vi "SS_PTF_indexer.vi"(6 "Faults Mod 5":bool[](array[boolean])=[FALSE, FALSE, FALSE], 8 "Faults Mod 4":bool[](array[boolean])=[FALSE, FALSE, FALSE], 9 "Faults Mod 3":bool[](array[boolean])=[FALSE, FALSE, FALSE, FALSE, FALSE, FALSE, FALSE, FALSE, FALSE, FALSE, FALSE, FALSE, FALSE, FALSE, FALSE, FALSE], 10 "Faults Mod 2":bool[](array[boolean])=[FALSE, FALSE, FALSE, FALSE, FALSE, FALSE, FALSE, FALSE, FALSE, FALSE, FALSE, FALSE, FALSE, FALSE, FALSE, FALSE], 11 "Faults Mod 1":bool[](array[boolean])=[FALSE, FALSE, FALSE, FALSE, FALSE, FALSE, FALSE, FALSE, FALSE, FALSE, FALSE, FALSE, FALSE, FALSE, FALSE, FALSE]) -> (3 "Group PTF":bool[](array[boolean]))   [LabVIEW 2016]
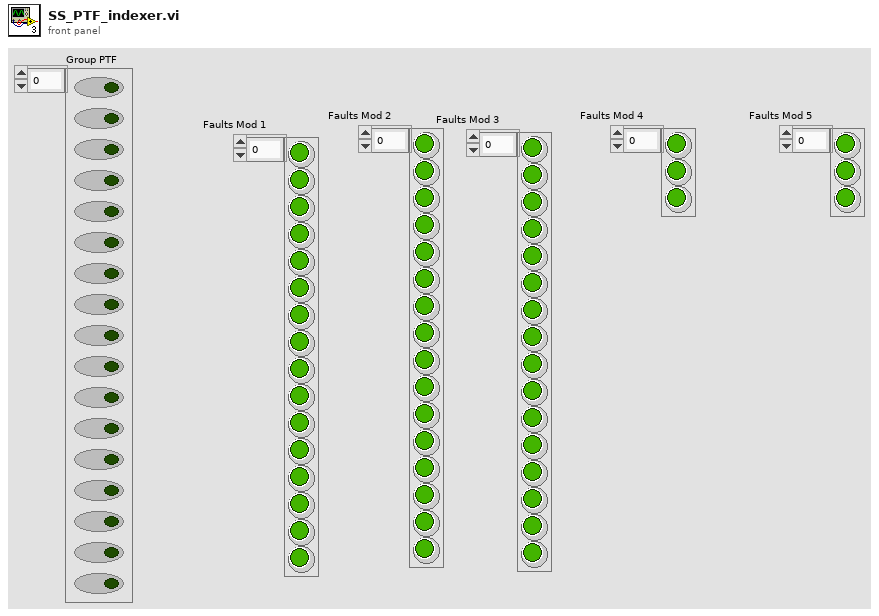
[diagram p1: front panel]
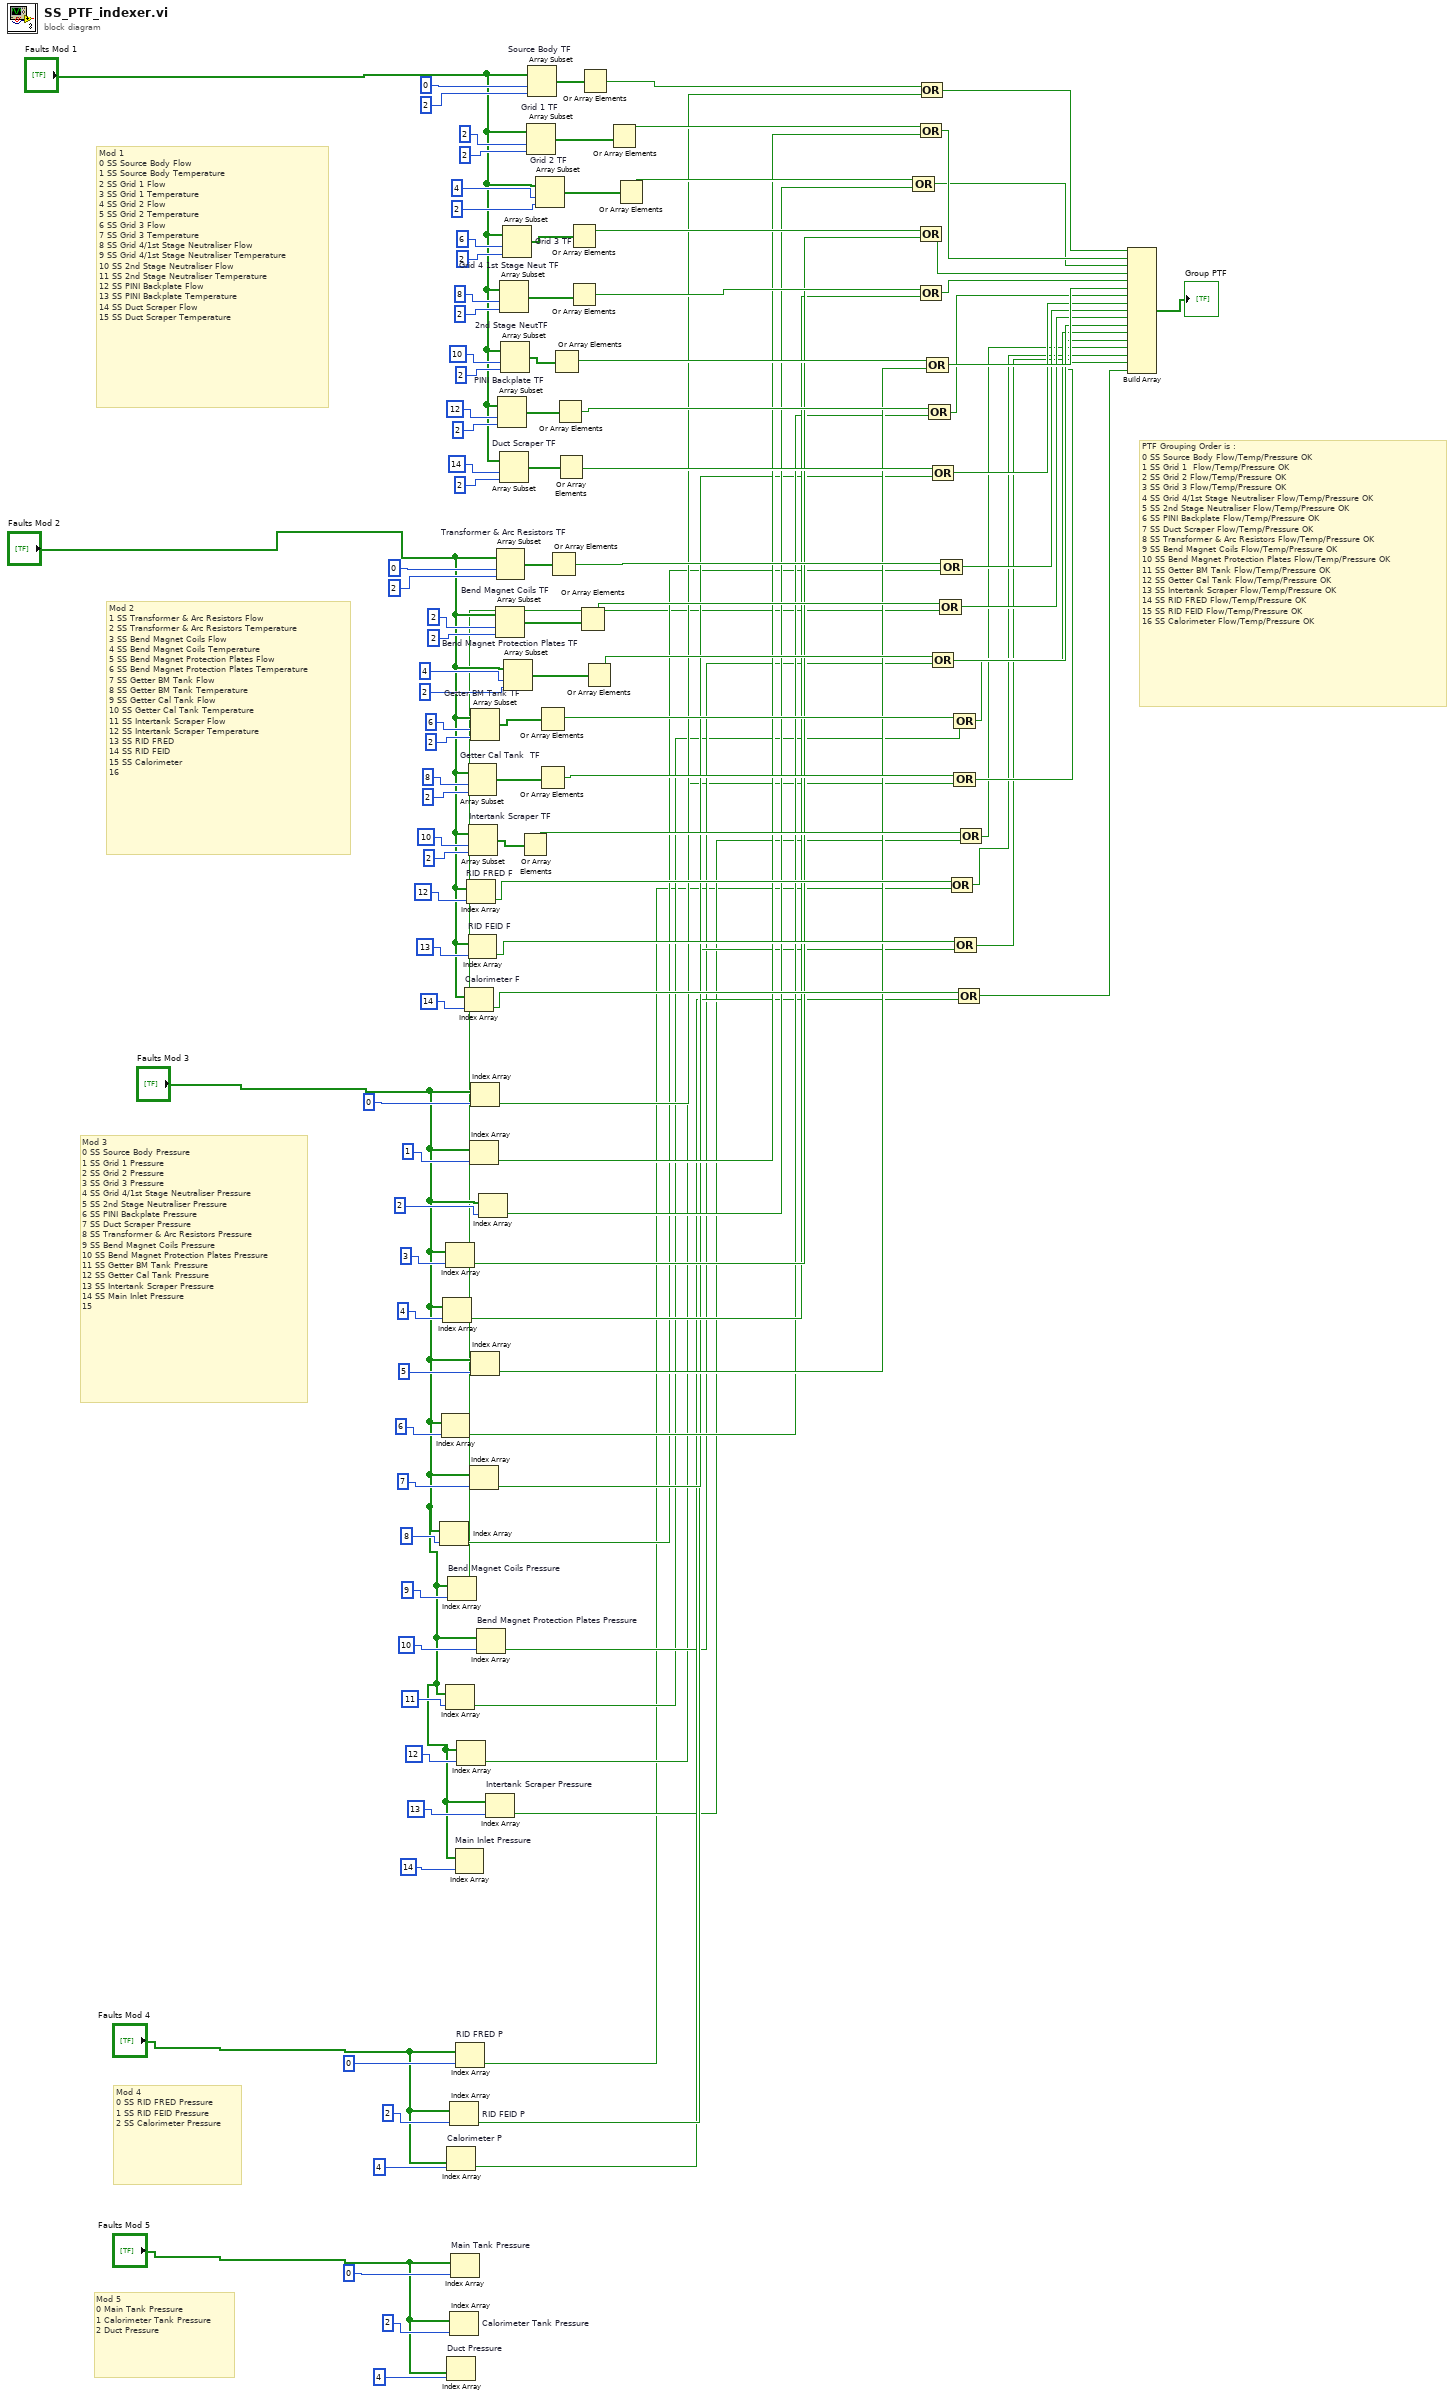
[diagram p0: block diagram]
diagram:
  # "Mod 5\n0\tMain Tank Pressure\n1\tCalorimeter Tank Pressure\n2\tDuct Pressure"
  # "Mod 4\n0\tSS RID FRED Pressure\n1\tSS RID FEID Pressure\n2\tSS Calorimeter Pressure"
  # "Mod 3\n0\tSS Source Body Pressure\n1\tSS Grid 1 Pressure\n2\tSS Grid 2 Pressure\n3\tSS Grid 3 Pressure\n4\tSS Grid 4/1st Stage Neutraliser Pressure\n5\tSS 2nd Stage Neutraliser Pressure\n6\tSS PINI Backplate Pressure\n7\tSS Duct Scraper Pressure\n8\tSS Transformer & Arc Resistors Pressure\n9\tSS Bend Magnet Coils Pressure\n10\tSS Bend Magnet Protection Plates Pressure\n11\tSS Getter BM Tank Pressure\n12\tSS Getter Cal Tank Pressure\n13\tSS Intertank Scraper Pressure\n14\tSS Main Inlet Pressure\n15"
  # "Mod 2\n1\tSS Transformer & Arc Resistors Flow\n2\tSS Transformer & Arc Resistors Temperature\n3\tSS Bend Magnet Coils Flow\n4\tSS Bend Magnet Coils Temperature\n5\tSS Bend Magnet Protection Plates Flow\n6\tSS Bend Magnet Protection Plates Temperature\n7\tSS Getter BM Tank Flow\n8\tSS Getter BM Tank Temperature\n9\tSS Getter Cal Tank Flow\n10\tSS Getter Cal Tank Temperature\n11\tSS Intertank Scraper Flow\n12\tSS Intertank Scraper Temperature\n13\tSS RID FRED\n14\tSS RID FEID\n15\tSS Calorimeter\n16"
  # "Mod 1\n0\tSS Source Body Flow\n1\tSS Source Body Temperature\n2\tSS Grid 1 Flow\n3\tSS Grid 1 Temperature\n4\tSS Grid 2 Flow\n5\tSS Grid 2 Temperature\n6\tSS Grid 3 Flow\n7\tSS Grid 3 Temperature\n8\tSS Grid 4/1st Stage Neutraliser Flow\n9\tSS Grid 4/1st Stage Neutraliser Temperature\n10\tSS 2nd Stage Neutraliser Flow\n11\tSS 2nd Stage Neutraliser Temperature\n12\tSS PINI Backplate Flow\n13\tSS PINI Backplate Temperature\n14\tSS Duct Scraper Flow\n15\tSS Duct Scraper Temperature"
  # "PTF Grouping Order is :\n0\tSS Source Body Flow/Temp/Pressure OK\n1\tSS Grid 1  Flow/Temp/Pressure OK\n2\tSS Grid 2 Flow/Temp/Pressure OK\n3\tSS Grid 3 Flow/Temp/Pressure OK\n4\tSS Grid 4/1st Stage Neutraliser Flow/Temp/Pressure OK\n5\tSS 2nd Stage Neutraliser Flow/Temp/Pressure OK\n6\tSS PINI Backplate Flow/Temp/Pressure OK\n7\tSS Duct Scraper Flow/Temp/Pressure OK\n8\tSS Transformer & Arc Resistors Flow/Temp/Pressure OK\n9\tSS Bend Magnet Coils Flow/Temp/Pressure OK\n10\tSS Bend Magnet Protection Plates Flow/Temp/Pressure OK\n11\tSS Getter BM Tank Flow/Temp/Pressure OK\n12\tSS Getter Cal Tank Flow/Temp/Pressure OK\n13\tSS Intertank Scraper Flow/Temp/Pressure OK\n14\tSS RID FRED Flow/Temp/Pressure OK\n15\tSS RID FEID Flow/Temp/Pressure OK\n16\tSS Calorimeter Flow/Temp/Pressure OK"
  n1 = Index Array "Index Array"(array="Faults Mod 3", index=8) -> (element=w25:bool)
  n2 = Index Array "Index Array"(array="Faults Mod 3", index=6) -> (element=w44:bool)
  n3 = Index Array "Index Array"(array="Faults Mod 3", index=4) -> (element=w46:bool)
  n4 = Index Array "Index Array"(array="Faults Mod 3", index=3) -> (element=w47:bool)
  n5 = Index Array "Index Array"(array="Faults Mod 3", index=11) -> (element=w22:bool)
  n6 = Index Array "Calorimeter P"(array="Faults Mod 4", index=4) -> (element=w37:bool)
  n7 = Index Array "Duct Pressure"(array="Faults Mod 5", index=4) -> ()  [unwired: 1 out]
  n8 = Index Array "Bend Magnet Coils Pressure"(array="Faults Mod 3", index=9) -> (element=w24:bool)
  n9 = Index Array "RID FEID P"(array="Faults Mod 4", index=2) -> (element=w38:bool)
  n10 = Index Array "Calorimeter Tank Pressure"(array="Faults Mod 5", index=2) -> ()  [unwired: 1 out]
  n11 = Index Array "Main Tank Pressure"(array="Faults Mod 5", index=0) -> ()  [unwired: 1 out]
  n12 = Index Array "Main Inlet Pressure"(array="Faults Mod 3", index=14) -> ()  [unwired: 1 out]
  n13 = Index Array "RID FRED P"(array="Faults Mod 4", index=0) -> (element=w19:bool)
  n14 = Index Array "Index Array"(array="Faults Mod 3", index=12) -> (element=w21:bool)
  n15 = Index Array "Calorimeter F"(array="Faults Mod 2", index=14) -> (element=w60:bool)
  n16 = Index Array "RID FRED F"(array="Faults Mod 2", index=12) -> (element=w61:bool)
  n17 = Array Subset "Getter Cal Tank  TF"(array="Faults Mod 2", index=8, length=2) -> (w73:bool[])
  n18 = Index Array "RID FEID F"(array="Faults Mod 2", index=13) -> (element=w62:bool)
  n19 = Array Subset "Intertank Scraper TF"(array="Faults Mod 2", index=10, length=2) -> (w74:bool[])
  n20 = Index Array "Index Array"(array="Faults Mod 3", index=1) -> (element=w49:bool)
  n21 = Index Array "Index Array"(array="Faults Mod 3", index=7) -> (element=w43:bool)
  n22 = Array Subset "Getter BM Tank TF"(array="Faults Mod 2", index=6, length=2) -> (w72:bool[])
  n23 = Index Array "Index Array"(array="Faults Mod 3", index=0) -> (element=w50:bool)
  n24 = Index Array "Index Array"(array="Faults Mod 3", index=5) -> (element=w45:bool)
  n25 = Index Array "Bend Magnet Protection Plates Pressure"(array="Faults Mod 3", index=10) -> (element=w23:bool)
  n26 = Index Array "Index Array"(array="Faults Mod 3", index=2) -> (element=w48:bool)
  n27 = Index Array "Intertank Scraper Pressure"(array="Faults Mod 3", index=13) -> (element=w20:bool)
  n28 = Array Subset "Bend Magnet Coils TF"(array="Faults Mod 2", index=2, length=2) -> (w70:bool[])
  n29 = Array Subset "Transformer & Arc Resistors TF"(array="Faults Mod 2", index=0, length=2) -> (w75:bool[])
  n30 = Array Subset "PINI Backplate TF"(array="Faults Mod 1", index=12, length=2) -> (w103:bool[])
  n31 = Array Subset "Grid 4 1st Stage Neut TF"(array="Faults Mod 1", index=8, length=2) -> (w101:bool[])
  n32 = Array Subset "Duct Scraper TF"(array="Faults Mod 1", index=14, length=2) -> (w104:bool[])
  n33 = Array Subset "2nd Stage NeutTF"(array="Faults Mod 1", index=10, length=2) -> (w102:bool[])
  n34 = Array Subset "Grid 3 TF"(array="Faults Mod 1", index=6, length=2) -> (w100:bool[])
  n35 = Array Subset "Bend Magnet Protection Plates TF"(array="Faults Mod 2", index=4, length=2) -> (w71:bool[])
  n36 = Or Array Elements(Boolean array=w74) -> (logical OR=w66:bool)
  n37 = Array Subset "Grid 1 TF"(array="Faults Mod 1", index=2, length=2) -> (w98:bool[])
  n38 = Array Subset "Source Body TF"(array="Faults Mod 1", index=0, length=2) -> (w105:bool[])
  n39 = Array Subset "Grid 2 TF"(array="Faults Mod 1", index=4, length=2) -> (w99:bool[])
  n40 = Or Array Elements(Boolean array=w72) -> (logical OR=w67:bool)
  n41 = Or Array Elements(Boolean array=w73) -> (logical OR=w65:bool)
  n42 = Or Array Elements(Boolean array=w75) -> (logical OR=w76:bool)
  n43 = Or Array Elements(Boolean array=w102) -> (logical OR=w94:bool)
  n44 = Or Array Elements(Boolean array=w103) -> (logical OR=w91:bool)
  n45 = Or Array Elements(Boolean array=w104) -> (logical OR=w93:bool)
  n46 = Or Array Elements(Boolean array=w100) -> (logical OR=w95:bool)
  n47 = Or Array Elements(Boolean array=w101) -> (logical OR=w92:bool)
  n48 = Or Array Elements(Boolean array=w70) -> (logical OR=w69:bool)
  n49 = Or Array Elements(Boolean array=w105) -> (logical OR=w106:bool)
  n50 = Or Array Elements(Boolean array=w71) -> (logical OR=w68:bool)
  n51 = Or Array Elements(Boolean array=w98) -> (logical OR=w97:bool)
  n52 = Or Array Elements(Boolean array=w99) -> (logical OR=w96:bool)
  n53 = Compound Arithmetic op=OR(w96, w48) -> (w16:bool)
  n54 = Compound Arithmetic op=OR(w97, w49) -> (w17:bool)
  n55 = Compound Arithmetic op=OR(w95, w47) -> (w15:bool)
  n56 = Compound Arithmetic op=OR(w92, w46) -> (w14:bool)
  n57 = Compound Arithmetic op=OR(w106, w50) -> (w18:bool)
  n58 = Compound Arithmetic op=OR(w94, w45) -> (w13:bool)
  n59 = Compound Arithmetic op=OR(w91, w44) -> (w12:bool)
  n60 = Compound Arithmetic op=OR(w93, w43) -> (w11:bool)
  n61 = Compound Arithmetic op=OR(w68, w23) -> (w8:bool)
  n62 = Compound Arithmetic op=OR(w69, w24) -> (w9:bool)
  n63 = Compound Arithmetic op=OR(w76, w25) -> (w10:bool)
  n64 = Compound Arithmetic op=OR(w61, w19) -> (w4:bool)
  n65 = Compound Arithmetic op=OR(w67, w22) -> (w7:bool)
  n66 = Compound Arithmetic op=OR(w65, w21) -> (w6:bool)
  n67 = Compound Arithmetic op=OR(w62, w38) -> (w3:bool)
  n68 = Compound Arithmetic op=OR(w60, w37) -> (w2:bool)
  n69 = Compound Arithmetic op=OR(w66, w20) -> (w5:bool)
  n70 = Build Array(w18, w17, w16, w15, w14, w13, w12, w11, w10, w9, w8, w7, w6, w5, w4, w3, w2) -> (→"Group PTF":bool[])
